vi "Mouse State FGV.vi"   [LabVIEW 2014]
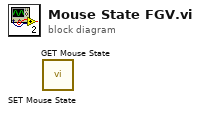
[diagram p0: block diagram]
diagram:
  n1 = call "SET Mouse State.vi"() -> ()  [unwired: 11 in, 1 out]
  n2 = call "GET Mouse State.vi"() -> ()  [unwired: 10 in, 2 out]
